vi "Get Error Controls.vi"(8 "error in (no error)":errorcluster, 10 "map":map{string, refnum<vi>}(c390), 11 "VI in":refnum<vi>) -> (0 "error out":errorcluster, 2 "map out":map{string, refnum<vi>}(c390), 3 "reference out":refnum<vi>)   [LabVIEW 2020, in "Mock Class Generator.lvclass"]
uses:
  Mock Class Generator.lvclass
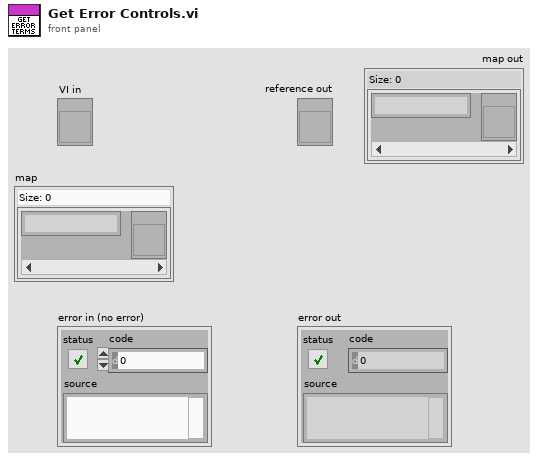
[diagram p1: front panel]
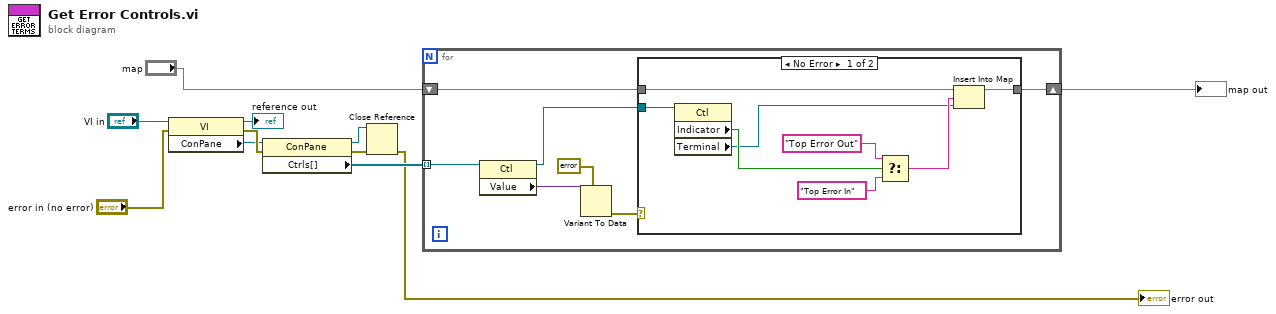
[diagram p0: block diagram]
diagram:
  n1 = property class="VI"(reference="VI in", error in="error in (no error)") -> (reference out=→"reference out":refnum<vi>, error out=w10:errorcluster, "ConPane"=w7:refnum<vi>)
  n2 = property class="ConPane"(reference=w7, error in=w10) -> (reference out=w4:refnum<vi>, error out=w9:errorcluster, "Ctrls[]"=w8:refnum<vi>[])
  n3 = Close Reference(reference=w4, error in (no error)=w9) -> (error out=→"error out":errorcluster)
  n4 = for {
    tunnel: w8 -> [w18] mode=indexing
    shift-right: [w14] -> w1
    shift-left: "map" -> [w15]
    n5 = property class="Ctl"(reference=w18) -> (reference out=w12:refnum<vi>, "Value"=w17:variant)  [unwired: 1 in, 1 out]
    n6 = Variant To Data(type=errorcluster {"status"=FALSE, "code"=0, "source"=""} ("error out"), Variant=w17) -> (error out=w13:errorcluster)  [unwired: 1 in, 1 out]
    n7 = case shown="No Error" w13 {
      tunnel: w15 -> [w26 w27]
      tunnel: [w25 w27] -> w14
      tunnel: w12 -> [w21 _]
      frame No Error {
        n8 = property class="Ctl"(reference=w21) -> ("Indicator"=w20:bool, "Terminal"=w19:refnum<vi>)  [unwired: 1 in, 2 out]
        n9 = Select(t="Top Error Out" ("key"), s=w20, f="Top Error In" ("key")) -> (s? t:f=w22:string)
        n10 = Insert Into Map(map in=w26, key=w22, value=w19) -> (map out=w25:map{string, refnum<vi>})  [unwired: 2 out]
      }
      frame Error {
      }
    }
  }
  "map out" <- w1
